vi "Drift_vec_plotting.vi"(0 "Application ref in":refnum<vi>, 2 "Plotting Data In":T1, 3 "error in":errorcluster) -> (5 "Application ref out":refnum<vi>, 6 "Vx vs. Scan #":picture, 7 "Vy vs. Scan #":picture, 8 "error out":errorcluster, 9 "Vz vs. Scan #":picture, 10 "Plotting Data Out":T1)   [LabVIEW 2025]
uses:
  <vilib>/picture/cartesn2.llb/XY Plot Type.ctl
  <userlib>/Nanonis Prog Interface V5/Nanonis Prog Interface.lvlib
panel:
  in  "cartesian axis attributes":T2={"x minimum"=0.0, "x maximum"=0.0, "x log?"=FALSE, "x precision"=1, "x format"=enum."Decimal", "y minimum"=-10000000000000.0, "y maximum"=1e-11, "y log?"=FALSE, "y precision"=1e-16, "y format"=enum."Scientific"} {"x minimum" format="%0.2f"; "x maximum" format="%0.2f"; "y minimum" format="%e"; "y maximum" format="%.16e"}
  in  "cartesian grid cosmetics":T3={"line color"=6710886, "text color"=13421772, "tick length(3)"=3, "crossing axes"=FALSE, "visible grid?"=TRUE}
  in  "XY plot cosmetics":T5={"plot color"=8388788, "XY plot type"=enum."connected squares", "baseline"=0.0} {"baseline" format="%0.2f"}
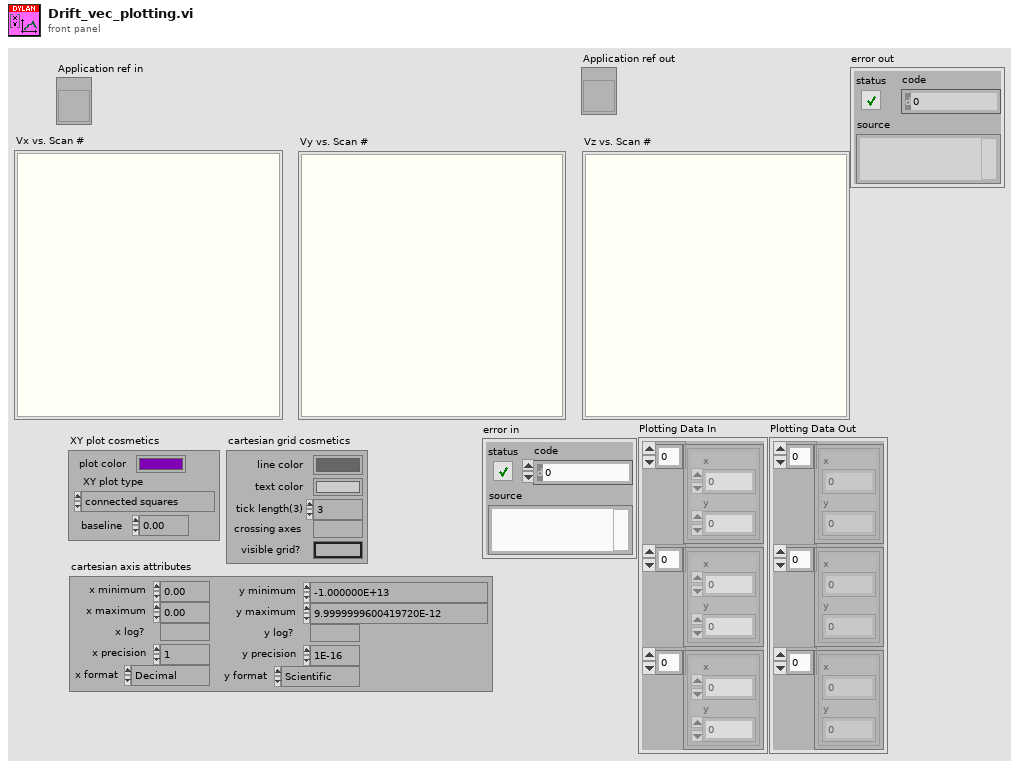
[diagram p1: front panel]
types:
  T1 = cluster{cluster{"x":sgl, "y":sgl}[], cluster{"x":sgl, "y":sgl}[], cluster{"x":sgl, "y":sgl}[]}
  T2 = cluster{"x minimum":dbl, "x maximum":dbl, "x log?":bool, "x precision":u8, "x format":enum8{"Decimal", "Scientific", "Engineering", "Binary", "Octal", "Hex"}, "y minimum":dbl, "y maximum":sgl, "y log?":bool, "y precision":sgl, "y format":enum8{"Decimal", "Scientific", "Engineering", "Binary", "Octal", "Hex"}}
  T3 = cluster{"line color":u32, "text color":u32, "tick length(3)":i16, "crossing axes":bool, "visible grid?":bool}
  T4 = typedef "XY Plot Type.ctl" = enum16{"points", "squares", "circles", "connected points", "connected squares", "connected circles", "comb plot", "sized scatter plot", "sized-colored scatter plot", "min-max lines"}
  T5 = cluster{"plot color":u32, "XY plot type":T4, "baseline":dbl}
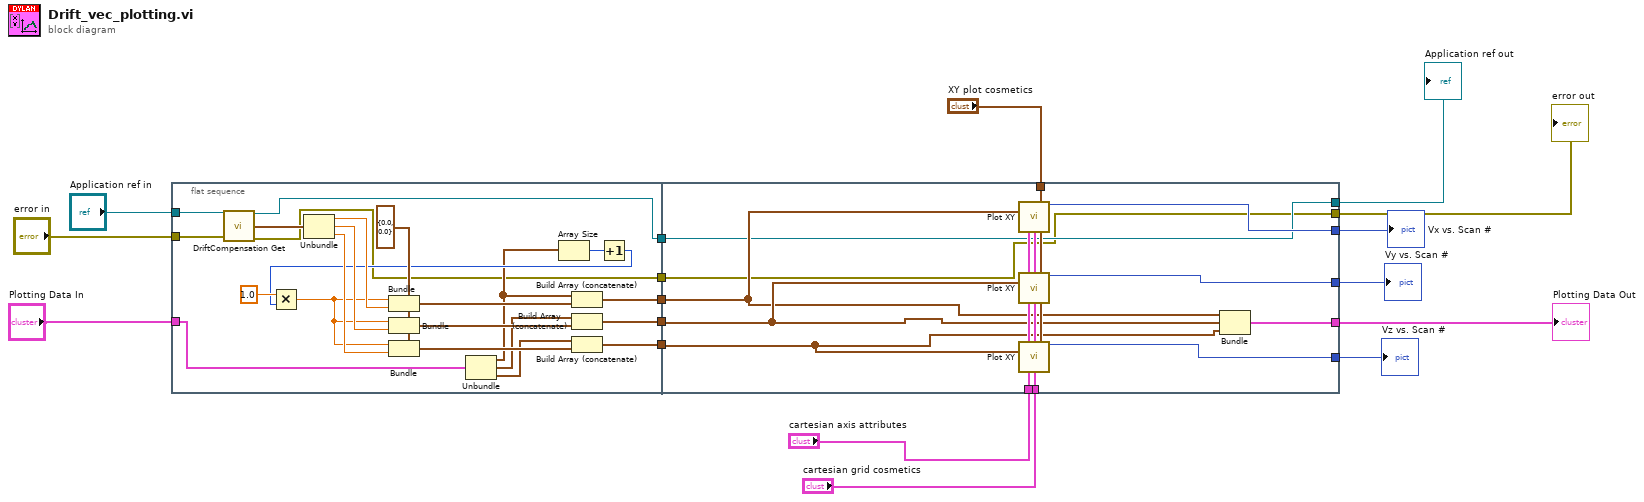
[diagram p0: block diagram]
diagram:
  n1 = flat-sequence {
    tunnel: "error in" -> [w39]
    tunnel: "Application ref in" -> [w40]
    tunnel: "Plotting Data In" -> [w21]
    tunnel: [w30] -> w17
    tunnel: [w29] -> w16
    tunnel: [w28] -> w15
    tunnel: [w19] -> w4
    tunnel: [w18] -> w3
    tunnel: w17 -> [w43]
    tunnel: w16 -> [w44]
    tunnel: w15 -> [w45]
    tunnel: "XY plot cosmetics" -> [w52]
    tunnel: [w51] -> w11
    tunnel: [w50] -> w10
    tunnel: [w49] -> w9
    tunnel: [w48] -> w5
    tunnel: "cartesian grid cosmetics" -> [w47]
    tunnel: "cartesian axis attributes" -> [w46]
    tunnel: [w42] -> w2
    tunnel: w4 -> [w42]
    tunnel: [w41] -> w1
    tunnel: w3 -> [w41]
    frame #0 {
      w37 = cluster{"x":sgl, "y":sgl} {"x"=0.0, "y"=0.0} ("Point [horizontal, vertical]")
      n2 = call <userlib>:"DriftCompensation Get.vi"("Application ref in"=w40, "error in (no error)"=w39) -> ("Application ref out"=w19:refnum<vi>, "Compensation speeds (m/s)"=w38:cluster{"Vx":sgl, "Vy":sgl, "Vz":sgl}, "error out"=w18:errorcluster)  [unwired: 8 in, 3 out]
      n3 = Unbundle(w38) -> ("Vx"=w36:sgl, "Vy"=w35:sgl, "Vz"=w34:sgl)
      n4 = Unbundle(w21) -> (w20:cluster{"x":sgl, "y":sgl}[], w25:cluster{"x":sgl, "y":sgl}[], w24:cluster{"x":sgl, "y":sgl}[])
      n5 = Array Size(array=w20) -> (size(s)=w23:i32)
      n6 = Increment(x=w23) -> (x+1=w22:i32)
      n7 = Multiply(x=sgl 1.0, y=w22) -> (x*y=w26:sgl)
      n8 = Bundle(cluster=w37, "x"=w26, "y"=w36) -> (w33:cluster{"x":sgl, "y":sgl})
      n9 = Bundle(cluster=w37, "x"=w26, "y"=w35) -> (w32:cluster{"x":sgl, "y":sgl})
      n10 = Bundle(cluster=w37, "x"=w26, "y"=w34) -> (w31:cluster{"x":sgl, "y":sgl})
      n11 = Build Array (concatenate)(w20, w33) -> (w30:cluster{"x":sgl, "y":sgl}[])
      n12 = Build Array (concatenate)(w25, w32) -> (w29:cluster{"x":sgl, "y":sgl}[])
      n13 = Build Array (concatenate)(w24, w31) -> (w28:cluster{"x":sgl, "y":sgl}[])
    }
    frame #1 {
      n14 = call <vilib>:"Plot XY.vi"("data"=w43, "cartesian axis attributes"=w46, "cartesian grid cosmetics"=w47, "XY plot cosmetics"=w52) -> ("new picture"=w51:picture)  [unwired: 11 in]
      n15 = call <vilib>:"Plot XY.vi"("data"=w44, "cartesian axis attributes"=w46, "cartesian grid cosmetics"=w47, "XY plot cosmetics"=w52) -> ("new picture"=w50:picture)  [unwired: 11 in]
      n16 = call <vilib>:"Plot XY.vi"("data"=w45, "cartesian axis attributes"=w46, "cartesian grid cosmetics"=w47, "XY plot cosmetics"=w52) -> ("new picture"=w49:picture)  [unwired: 11 in]
      n17 = Bundle(w43, w44, w45) -> (w48:T1)  [unwired: 1 in]
    }
  }
  "Vx vs. Scan #" <- w11
  "Vy vs. Scan #" <- w10
  "Vz vs. Scan #" <- w9
  "Plotting Data Out" <- w5
  "Application ref out" <- w2
  "error out" <- w1
